vi "Basic DMA.vi"() -> ()   [LabVIEW 2023]
doc: "This basic example shows sending data to the FPGA and back to the host via DMA transfers to verify proper board operation."
uses:
  <vilib>/userDefined/Silver/nirio_resource_slv.ctl
  <vilib>/FPGAPlugInAG/PXIe-7915/niLvFpga_Open_PXIe-7915.vi
  <vilib>/rvi/interface/common/dynamic/niFpgaDynamicAddResources.vi
  <vilib>/Utility/error.llb/Error Cluster From Error Code.vi
  <vilib>/rvi/errors/niLvFpgaAdjustHostInterfaceError.vi
  <vilib>/FPGAPlugInAG/Dynamic/niLvFpga_Close_Dynamic.vi
  <vilib>/rvi/interface/nirviOpenFPGA/nirviOpenFPGA.xnode
  FPGA Bitfiles/PXIe-791X_Getting_Started.lvbitx
  <vilib>/rvi/interface/nirviReadWriteControl/nirviReadWriteControl.xnode
  <vilib>/rvi/interface/nirviMethod/nirviMethod.xnode
  <vilib>/rvi/interface/nirviCloseFPGA/nirviCloseFPGA.xnode
  <vilib>/measure/NI_MABase.lvlib
  <instrlib>/_niInstr/Streaming/v1/Host/niInstr Streaming v1 Host.lvlib
  <vilib>/rvi/errors/niLvFpgaMergeErrorWithErrorCode.vi
  NiFpgaLv.dll
  <vilib>/rvi/interface/Simulation/niFpgaSimulationCallBeginRW.vi
  <vilib>/FPGAPlugInAG/Dynamic/niLvFpga_WriteFifo_Dynamic.vi
  <vilib>/FPGAPlugInAG/Dynamic/niLvFpga_ReadFifo_Dynamic.vi
panel:
  out "Signal In":i16[](graph)=[0, 655, 1311, 1966, 2621, 3277, 3932, 4587, 5243, 5898, 6553, 7209, 7864, 8519, 9175, 9830, 10485, 11141, 11796, 12451, 13107, 13762, 14417, 15073, 15728, 16384, 17039, 17694, 18350, 19005, 19660, 20316, 20971, 21626, 22282, 22937, 23592, 24248, 24903, 25558, 26214, 26869, 27524, 28180, 28835, 29490, 30146, 30801, 31456, 32112, -32767, -32112, -31456, -30801, -30146, -29490, -28835, -28180, -27524, -26869, -26214, -25558, -24903, -24248, -23592, -22937, -22282, -21626, -20971, -20316, -19660, -19005, -18350, -17694, -17039, -16384, -15728, -15073, -14417, -13762, -13107, -12451, -11796, -11141, -10485, -9830, -9175, -8519, -7864, -7209, -6553, -5898, -5243, -4587, -3932, -3277, -2621, -1966, -1311, -655, 0, 655, 1311, 1966, 2621, 3277, 3932, 4587, 5243, 5898, 6553, 7209, 7864, 8519, 9175, 9830, 10485, 11141, 11796, 12451, 13107, 13762, 14417, 15073, 15728, 16384, 17039, 17694, 18350, 19005, 19660, 20316, 20971, 21626, 22282, 22937, 23592, 24248, 24903, 25558, 26214, 26869, 27524, 28180, 28835, 29490, 30146, 30801, 31456, 32112, -32767, -32112, -31456, -30801, -30146, -29490, -28835, -28180, -27524, -26869, -26214, -25558, -24903, -24248, -23592, -22937, -22282, -21626, -20971, -20316, -19660, -19005, -18350, -17694, -17039, -16384, -15728, -15073, -14417, -13762, -13107, -12451, -11796, -11141, -10485, -9830, -9175, -8519, -7864, -7209, -6553, -5898, -5243, -4587, -3932, -3277, -2621, -1966, -1311, -655, 0, 655, 1311, 1966, 2621, 3277, 3932, 4587, 5243, 5898, 6553, 7209, 7864, 8519, 9175, 9830, 10485, 11141, 11796, 12451, 13107, 13762, 14417, 15073, 15728, 16384, 17039, 17694, 18350, 19005, 19660, 20316, 20971, 21626, 22282, 22937, 23592, 24248, 24903, 25558, 26214, 26869, 27524, 28180, 28835, 29490, 30146, 30801, 31456, 32112, -32767, -32112, -31456, -30801, -30146, -29490, -28835, -28180, -27524, -26869, -26214, -25558, -24903, -24248, -23592, -22937, -22282, -21626, -20971, -20316, -19660, -19005, -18350, -17694, -17039, -16384, -15728, -15073, -14417, -13762, -13107, -12451, -11796, -11141, -10485, -9830, -9175, -8519, -7864, -7209, -6553, -5898, -5243, -4587, -3932, -3277, -2621, -1966, -1311, -655, 0, 655, 1311, 1966, 2621, 3277, 3932, 4587, 5243, 5898, 6553, 7209, 7864, 8519, 9175, 9830, 10485, 11141, 11796, 12451, 13107, 13762, 14417, 15073, 15728, 16384, 17039, 17694, 18350, 19005, 19660, 20316, 20971, 21626, 22282, 22937, 23592, 24248, 24903, 25558, 26214, 26869, 27524, 28180, 28835, 29490, 30146, 30801, 31456, 32112, -32767, -32112, -31456, -30801, -30146, -29490, -28835, -28180, -27524, -26869, -26214, -25558, -24903, -24248, -23592, -22937, -22282, -21626, -20971, -20316, -19660, -19005, -18350, -17694, -17039, -16384, -15728, -15073, -14417, -13762, -13107, -12451, -11796, -11141, -10485, -9830, -9175, -8519, -7864, -7209, -6553, -5898, -5243, -4587, -3932, -3277, -2621, -1966, -1311, -655, 0, 655, 1311, 1966, 2621, 3277, 3932, 4587, 5243, 5898, 6553, 7209, 7864, 8519, 9175, 9830, 10485, 11141, 11796, 12451, 13107, 13762, 14417, 15073, 15728, 16384, 17039, 17694, 18350, 19005, 19660, 20316, 20971, 21626, 22282, 22937, 23592, 24248, 24903, 25558, 26214, 26869, 27524, 28180, 28835, 29490, 30146, 30801, 31456, 32112, -32767, -32112, -31456, -30801, -30146, -29490, -28835, -28180, -27524, -26869, -26214, -25558, -24903, -24248, -23592, -22937, -22282, -21626, -20971, -20316, -19660, -19005, -18350, -17694, -17039, -16384, -15728, -15073, -14417, -13762, -13107, -12451, -11796, -11141, -10485, -9830, -9175, -8519, -7864, -7209, -6553, -5898, -5243, -4587, -3932, -3277, -2621, -1966, -1311, -655, 0, 655, 1311, 1966, 2621, 3277, 3932, 4587, 5243, 5898, 6553, 7209, 7864, 8519, 9175, 9830, 10485, 11141, 11796, 12451, 13107, 13762, 14417, 15073, 15728, 16384, 17039, 17694, 18350, 19005, 19660, 20316, 20971, 21626, 22282, 22937, 23592, 24248, 24903, 25558, 26214, 26869, 27524, 28180, 28835, 29490, 30146, 30801, 31456, 32112, -32767, -32112, -31456, -30801, -30146, -29490, -28835, -28180, -27524, -26869, -26214, -25558, -24903, -24248, -23592, -22937, -22282, -21626, -20971, -20316, -19660, -19005, -18350, -17694, -17039, -16384, -15728, -15073, -14417, -13762, -13107, -12451, -11796, -11141, -10485, -9830, -9175, -8519, -7864, -7209, -6553, -5898, -5243, -4587, -3932, -3277, -2621, -1966, -1311, -655, 0, 655, 1311, 1966, 2621, 3277, 3932, 4587, 5243, 5898, 6553, 7209, 7864, 8519, 9175, 9830, 10485, 11141, 11796, 12451, 13107, 13762, 14417, 15073, 15728, 16384, 17039, 17694, 18350, 19005, 19660, 20316, 20971, 21626, 22282, 22937, 23592, 24248, 24903, 25558, 26214, 26869, 27524, 28180, 28835, 29490, 30146, 30801, 31456, 32112, -32767, -32112, -31456, -30801, -30146, -29490, -28835, -28180, -27524, -26869, -26214, -25558, -24903, -24248, -23592, -22937, -22282, -21626, -20971, -20316, -19660, -19005, -18350, -17694, -17039, -16384, -15728, -15073, -14417, -13762, -13107, -12451, -11796, -11141, -10485, -9830, -9175, -8519, -7864, -7209, -6553, -5898, -5243, -4587, -3932, -3277, -2621, -1966, -1311, -655, 0, 655, 1311, 1966, 2621, 3277, 3932, 4587, 5243, 5898, 6553, 7209, 7864, 8519, 9175, 9830, 10485, 11141, 11796, 12451, 13107, 13762, 14417, 15073, 15728, 16384, 17039, 17694, 18350, 19005, 19660, 20316, 20971, 21626, 22282, 22937, 23592, 24248, 24903, 25558, 26214, 26869, 27524, 28180, 28835, 29490, 30146, 30801, 31456, 32112, -32767, -32112, -31456, -30801, -30146, -29490, -28835, -28180, -27524, -26869, -26214, -25558, -24903, -24248, -23592, -22937, -22282, -21626, -20971, -20316, -19660, -19005, -18350, -17694, -17039, -16384, -15728, -15073, -14417, -13762, -13107, -12451, -11796, -11141, -10485, -9830, -9175, -8519, -7864, -7209, -6553, -5898, -5243, -4587, -3932, -3277, -2621, -1966, -1311, -655, 0, 655, 1311, 1966, 2621, 3277, 3932, 4587, 5243, 5898, 6553, 7209, 7864, 8519, 9175, 9830, 10485, 11141, 11796, 12451, 13107, 13762, 14417, 15073, 15728, 16384, 17039, 17694, 18350, 19005, 19660, 20316, 20971, 21626, 22282, 22937, 23592, 24248, 24903, 25558, 26214, 26869, 27524, 28180, 28835, 29490, 30146, 30801, 31456, 32112, -32767, -32112, -31456, -30801, -30146, -29490, -28835, -28180, -27524, -26869, -26214, -25558, -24903, -24248, -23592, -22937, -22282, -21626, -20971, -20316, -19660, -19005, -18350, -17694, -17039, -16384, -15728, -15073, -14417, -13762, -13107, -12451, -11796, -11141, -10485, -9830, -9175, -8519, -7864, -7209, -6553, -5898, -5243, -4587, -3932, -3277, -2621, -1966, -1311, -655, 0, 655, 1311, 1966, 2621, 3277, 3932, 4587, 5243, 5898, 6553, 7209, 7864, 8519, 9175, 9830, 10485, 11141, 11796, 12451, 13107, 13762, 14417, 15073, 15728, 16384, 17039, 17694, 18350, 19005, 19660, 20316, 20971, 21626, 22282, 22937, 23592, 24248, 24903, 25558, 26214, 26869, 27524, 28180, 28835, 29490, 30146, 30801, 31456, 32112, -32767, -32112, -31456, -30801, -30146, -29490, -28835, -28180, -27524, -26869, -26214, -25558, -24903, -24248, -23592, -22937, -22282, -21626, -20971, -20316, -19660, -19005, -18350, -17694, -17039, -16384, -15728, -15073, -14417, -13762, -13107, -12451, -11796, -11141, -10485, -9830, -9175, -8519, -7864, -7209, -6553, -5898, -5243, -4587, -3932, -3277, -2621, -1966, -1311, -655]
  out "Signal Out":i16[](graph)=[0, 655, 1311, 1966, 2621, 3277, 3932, 4587, 5243, 5898, 6553, 7209, 7864, 8519, 9175, 9830, 10485, 11141, 11796, 12451, 13107, 13762, 14417, 15073, 15728, 16384, 17039, 17694, 18350, 19005, 19660, 20316, 20971, 21626, 22282, 22937, 23592, 24248, 24903, 25558, 26214, 26869, 27524, 28180, 28835, 29490, 30146, 30801, 31456, 32112, -32767, -32112, -31456, -30801, -30146, -29490, -28835, -28180, -27524, -26869, -26214, -25558, -24903, -24248, -23592, -22937, -22282, -21626, -20971, -20316, -19660, -19005, -18350, -17694, -17039, -16384, -15728, -15073, -14417, -13762, -13107, -12451, -11796, -11141, -10485, -9830, -9175, -8519, -7864, -7209, -6553, -5898, -5243, -4587, -3932, -3277, -2621, -1966, -1311, -655, 0, 655, 1311, 1966, 2621, 3277, 3932, 4587, 5243, 5898, 6553, 7209, 7864, 8519, 9175, 9830, 10485, 11141, 11796, 12451, 13107, 13762, 14417, 15073, 15728, 16384, 17039, 17694, 18350, 19005, 19660, 20316, 20971, 21626, 22282, 22937, 23592, 24248, 24903, 25558, 26214, 26869, 27524, 28180, 28835, 29490, 30146, 30801, 31456, 32112, -32767, -32112, -31456, -30801, -30146, -29490, -28835, -28180, -27524, -26869, -26214, -25558, -24903, -24248, -23592, -22937, -22282, -21626, -20971, -20316, -19660, -19005, -18350, -17694, -17039, -16384, -15728, -15073, -14417, -13762, -13107, -12451, -11796, -11141, -10485, -9830, -9175, -8519, -7864, -7209, -6553, -5898, -5243, -4587, -3932, -3277, -2621, -1966, -1311, -655, 0, 655, 1311, 1966, 2621, 3277, 3932, 4587, 5243, 5898, 6553, 7209, 7864, 8519, 9175, 9830, 10485, 11141, 11796, 12451, 13107, 13762, 14417, 15073, 15728, 16384, 17039, 17694, 18350, 19005, 19660, 20316, 20971, 21626, 22282, 22937, 23592, 24248, 24903, 25558, 26214, 26869, 27524, 28180, 28835, 29490, 30146, 30801, 31456, 32112, -32767, -32112, -31456, -30801, -30146, -29490, -28835, -28180, -27524, -26869, -26214, -25558, -24903, -24248, -23592, -22937, -22282, -21626, -20971, -20316, -19660, -19005, -18350, -17694, -17039, -16384, -15728, -15073, -14417, -13762, -13107, -12451, -11796, -11141, -10485, -9830, -9175, -8519, -7864, -7209, -6553, -5898, -5243, -4587, -3932, -3277, -2621, -1966, -1311, -655, 0, 655, 1311, 1966, 2621, 3277, 3932, 4587, 5243, 5898, 6553, 7209, 7864, 8519, 9175, 9830, 10485, 11141, 11796, 12451, 13107, 13762, 14417, 15073, 15728, 16384, 17039, 17694, 18350, 19005, 19660, 20316, 20971, 21626, 22282, 22937, 23592, 24248, 24903, 25558, 26214, 26869, 27524, 28180, 28835, 29490, 30146, 30801, 31456, 32112, -32767, -32112, -31456, -30801, -30146, -29490, -28835, -28180, -27524, -26869, -26214, -25558, -24903, -24248, -23592, -22937, -22282, -21626, -20971, -20316, -19660, -19005, -18350, -17694, -17039, -16384, -15728, -15073, -14417, -13762, -13107, -12451, -11796, -11141, -10485, -9830, -9175, -8519, -7864, -7209, -6553, -5898, -5243, -4587, -3932, -3277, -2621, -1966, -1311, -655, 0, 655, 1311, 1966, 2621, 3277, 3932, 4587, 5243, 5898, 6553, 7209, 7864, 8519, 9175, 9830, 10485, 11141, 11796, 12451, 13107, 13762, 14417, 15073, 15728, 16384, 17039, 17694, 18350, 19005, 19660, 20316, 20971, 21626, 22282, 22937, 23592, 24248, 24903, 25558, 26214, 26869, 27524, 28180, 28835, 29490, 30146, 30801, 31456, 32112, -32767, -32112, -31456, -30801, -30146, -29490, -28835, -28180, -27524, -26869, -26214, -25558, -24903, -24248, -23592, -22937, -22282, -21626, -20971, -20316, -19660, -19005, -18350, -17694, -17039, -16384, -15728, -15073, -14417, -13762, -13107, -12451, -11796, -11141, -10485, -9830, -9175, -8519, -7864, -7209, -6553, -5898, -5243, -4587, -3932, -3277, -2621, -1966, -1311, -655, 0, 655, 1311, 1966, 2621, 3277, 3932, 4587, 5243, 5898, 6553, 7209, 7864, 8519, 9175, 9830, 10485, 11141, 11796, 12451, 13107, 13762, 14417, 15073, 15728, 16384, 17039, 17694, 18350, 19005, 19660, 20316, 20971, 21626, 22282, 22937, 23592, 24248, 24903, 25558, 26214, 26869, 27524, 28180, 28835, 29490, 30146, 30801, 31456, 32112, -32767, -32112, -31456, -30801, -30146, -29490, -28835, -28180, -27524, -26869, -26214, -25558, -24903, -24248, -23592, -22937, -22282, -21626, -20971, -20316, -19660, -19005, -18350, -17694, -17039, -16384, -15728, -15073, -14417, -13762, -13107, -12451, -11796, -11141, -10485, -9830, -9175, -8519, -7864, -7209, -6553, -5898, -5243, -4587, -3932, -3277, -2621, -1966, -1311, -655, 0, 655, 1311, 1966, 2621, 3277, 3932, 4587, 5243, 5898, 6553, 7209, 7864, 8519, 9175, 9830, 10485, 11141, 11796, 12451, 13107, 13762, 14417, 15073, 15728, 16384, 17039, 17694, 18350, 19005, 19660, 20316, 20971, 21626, 22282, 22937, 23592, 24248, 24903, 25558, 26214, 26869, 27524, 28180, 28835, 29490, 30146, 30801, 31456, 32112, -32767, -32112, -31456, -30801, -30146, -29490, -28835, -28180, -27524, -26869, -26214, -25558, -24903, -24248, -23592, -22937, -22282, -21626, -20971, -20316, -19660, -19005, -18350, -17694, -17039, -16384, -15728, -15073, -14417, -13762, -13107, -12451, -11796, -11141, -10485, -9830, -9175, -8519, -7864, -7209, -6553, -5898, -5243, -4587, -3932, -3277, -2621, -1966, -1311, -655, 0, 655, 1311, 1966, 2621, 3277, 3932, 4587, 5243, 5898, 6553, 7209, 7864, 8519, 9175, 9830, 10485, 11141, 11796, 12451, 13107, 13762, 14417, 15073, 15728, 16384, 17039, 17694, 18350, 19005, 19660, 20316, 20971, 21626, 22282, 22937, 23592, 24248, 24903, 25558, 26214, 26869, 27524, 28180, 28835, 29490, 30146, 30801, 31456, 32112, -32767, -32112, -31456, -30801, -30146, -29490, -28835, -28180, -27524, -26869, -26214, -25558, -24903, -24248, -23592, -22937, -22282, -21626, -20971, -20316, -19660, -19005, -18350, -17694, -17039, -16384, -15728, -15073, -14417, -13762, -13107, -12451, -11796, -11141, -10485, -9830, -9175, -8519, -7864, -7209, -6553, -5898, -5243, -4587, -3932, -3277, -2621, -1966, -1311, -655, 0, 655, 1311, 1966, 2621, 3277, 3932, 4587, 5243, 5898, 6553, 7209, 7864, 8519, 9175, 9830, 10485, 11141, 11796, 12451, 13107, 13762, 14417, 15073, 15728, 16384, 17039, 17694, 18350, 19005, 19660, 20316, 20971, 21626, 22282, 22937, 23592, 24248, 24903, 25558, 26214, 26869, 27524, 28180, 28835, 29490, 30146, 30801, 31456, 32112, -32767, -32112, -31456, -30801, -30146, -29490, -28835, -28180, -27524, -26869, -26214, -25558, -24903, -24248, -23592, -22937, -22282, -21626, -20971, -20316, -19660, -19005, -18350, -17694, -17039, -16384, -15728, -15073, -14417, -13762, -13107, -12451, -11796, -11141, -10485, -9830, -9175, -8519, -7864, -7209, -6553, -5898, -5243, -4587, -3932, -3277, -2621, -1966, -1311, -655, 0, 655, 1311, 1966, 2621, 3277, 3932, 4587, 5243, 5898, 6553, 7209, 7864, 8519, 9175, 9830, 10485, 11141, 11796, 12451, 13107, 13762, 14417, 15073, 15728, 16384, 17039, 17694, 18350, 19005, 19660, 20316, 20971, 21626, 22282, 22937, 23592, 24248, 24903, 25558, 26214, 26869, 27524, 28180, 28835, 29490, 30146, 30801, 31456, 32112, -32767, -32112, -31456, -30801, -30146, -29490, -28835, -28180, -27524, -26869, -26214, -25558, -24903, -24248, -23592, -22937, -22282, -21626, -20971, -20316, -19660, -19005, -18350, -17694, -17039, -16384, -15728, -15073, -14417, -13762, -13107, -12451, -11796, -11141, -10485, -9830, -9175, -8519, -7864, -7209, -6553, -5898, -5243, -4587, -3932, -3277, -2621, -1966, -1311, -655]
  in  "Simulated Signal Type":T1(ring)=enum."Sawtooth Wave"
  in  "791x Resource":T2="RIO0"
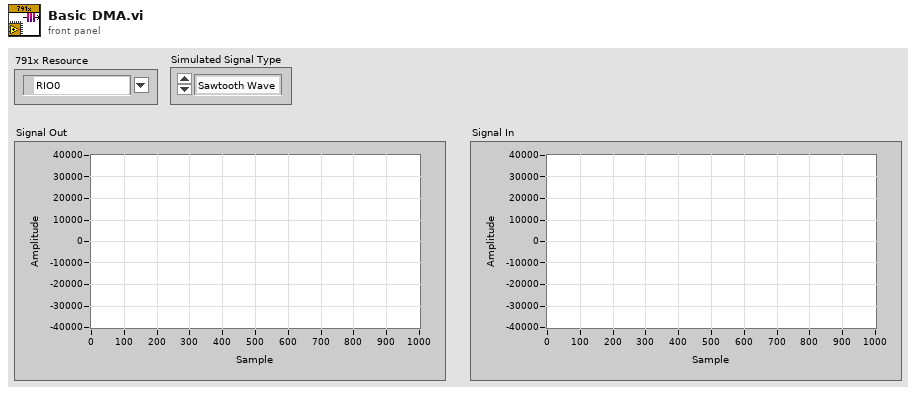
[diagram p1: front panel]
types:
  T1 = enum16{"Sine Wave", "Triangle Wave", "Square Wave", "Sawtooth Wave"}
  T2 = typedef "nirio_resource_slv.ctl" = tag
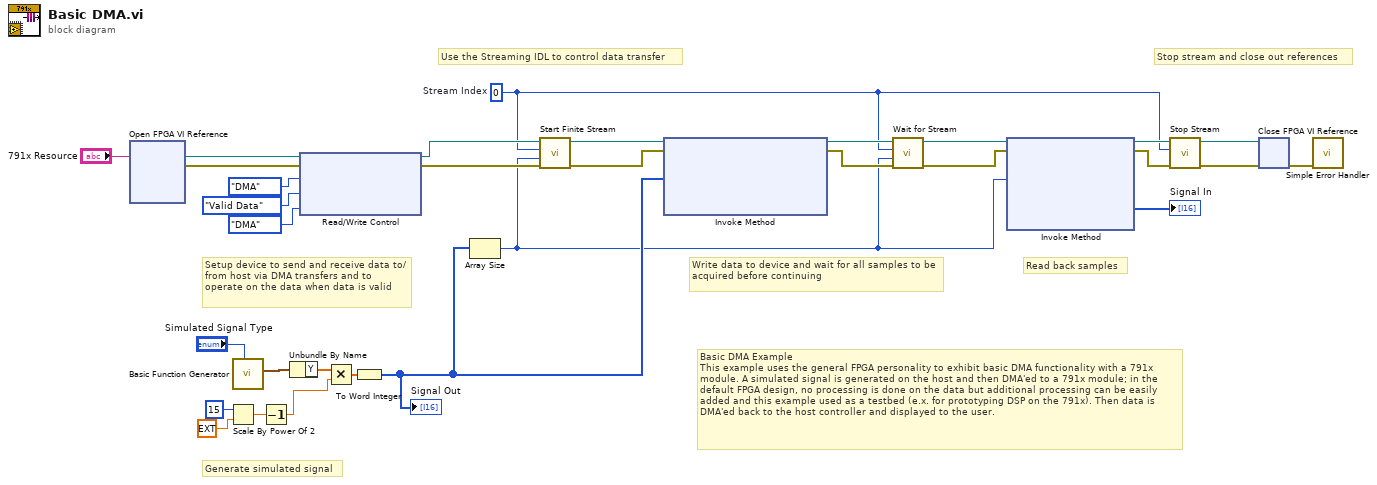
[diagram p0: block diagram]
diagram:
  w4 = 0  # Stream Index
  # "Basic DMA Example\nThis example uses the general FPGA personality to exhibit basic DMA functionality with a 791x module. A simulated signal is generated on the host and then DMA'ed to a 791x module; in the default FPGA design, no processing is done on the data but additional processing can be easily added and this example used as a testbed (e.x. for prototyping DSP on the 791x). Then data is DMA'ed back to the host controller and displayed to the user."
  # "Stop stream and close out references"
  # "Read back samples"
  # "Write data to device and wait for all samples to be acquired before continuing"
  # "Use the Streaming IDL to control data transfer"
  # "Generate simulated signal"
  # "Setup device to send and receive data to/from host via DMA transfers and to operate on the data when data is valid"
  n1 = xnode "Open FPGA VI Reference"("resource name"="791x Resource") -> ("FPGA VI Reference Out"=w22:refnum<k20>, "error out"=w21:errorcluster)  [unwired: 1 in]
  n2 = Scale By Power Of 2(n=i16 15, x=ext 1.0) -> (x*2^n=w28:ext)
  n3 = call <vilib>:"Basic Function Generator.vi"("signal type"="Simulated Signal Type") -> ("signal out"=w27:waveform(dbl))  [unwired: 8 in, 2 out]
  n4 = Decrement(x=w28) -> (x-1=w25:ext)
  n5 = Unbundle By Name(w27) -> ("Y"=w26:dbl[])
  n6 = xnode "Read/Write Control"("FPGA VI Reference In"=w22, "error in"=w21, "Data Source"=enum16{"DMA", "P2P"}."DMA", "Data Source Trigger"=enum16{"Valid Data", "Software"}."Valid Data", "Data Sink"=enum16{"DMA", "P2P"}."DMA") -> ("FPGA VI Reference Out"=w16:refnum<k20>, "error out"=w17:errorcluster)
  n7 = Multiply(x=w26, y=w25) -> (x*y=w24:ext[])
  n8 = To Word Integer(number=w24) -> (16bit integer=w13:i16[])
  "Signal Out" <- w13
  n9 = Array Size(array=w13) -> (size(s)=w8:i32)
  n10 = call <instrlib>:"Start Finite Stream.vi"("error in (no error)"=w17, "num samples"=w8, "stream index"=w4, "refnum in"=w16) -> ("error out"=w14:errorcluster, "refnum out"=w15:refnum<k20>)  [unwired: 6 in]
  n11 = xnode "Invoke Method"("FPGA VI Reference In"=w15, "error in"=w14, "Data"=w13) -> ("FPGA VI Reference Out"=w12:refnum<k20>, "error out"=w11:errorcluster)  [unwired: 1 in, 1 out]
  n12 = call <instrlib>:"Wait for Stream.vi"("error in (no error)"=w11, "wait for samples transferred"=w8, "stream index"=w4, "refnum in"=w12) -> ("error out"=w9:errorcluster, "refnum out"=w10:refnum<k20>)  [unwired: 4 in, 2 out]
  n13 = xnode "Invoke Method"("FPGA VI Reference In"=w10, "error in"=w9, "Number of Elements"=w8) -> ("FPGA VI Reference Out"=w6:refnum<k20>, "error out"=w5:errorcluster, "Data"=→"Signal In":i16[])  [unwired: 1 in, 1 out]
  n14 = call <instrlib>:"Stop Stream.vi"("error in (no error)"=w5, "stream index"=w4, "refnum in"=w6) -> ("error out"=w3:errorcluster, "refnum out"=w2:refnum<k20>)  [unwired: 5 in, 2 out]
  n15 = xnode "Close FPGA VI Reference"("FPGA VI Reference In"=w2, "error in"=w3) -> ("error out"=w1:errorcluster)
  n16 = call <vilib>:"Simple Error Handler.vi"("error in (no error)"=w1) -> ()  [unwired: 4 in, 5 out]
